vi "JSON DATA.vi"(0 "Temp Amb":refnum<class "JSON Object.lvclass">[](array[class]), 1 "Humedad R.":refnum<class "JSON Object.lvclass">[](array[class]), 2 "PAR":refnum<class "JSON Object.lvclass">[](array[class]), 3 "Numeric":i32, 5 "Temp Panel":refnum<class "JSON Object.lvclass">[](array[class]), 7 "Generador":refnum<class "JSON Object.lvclass">[](array[class]), 9 "JSON CARGA":refnum<class "JSON Array.lvclass">[](array[class]), 11 "error in":errorcluster, 12 "JSON FV":refnum<class "JSON Object.lvclass">[](array[class]), 13 "JSON BAT":refnum<class "JSON Object.lvclass">[](array[class]), 14 "alarmas":refnum<class "JSON Array.lvclass">[](array[class])) -> (4 "Array":refnum<class "JSON Object.lvclass">[](array[class]), 15 "error out":errorcluster)   [LabVIEW 2015]
uses:
  <vilib>/addons/JSON API/JSON Object/JSON Object.lvclass
  <vilib>/addons/JSON API/JSON Array/JSON Array.lvclass
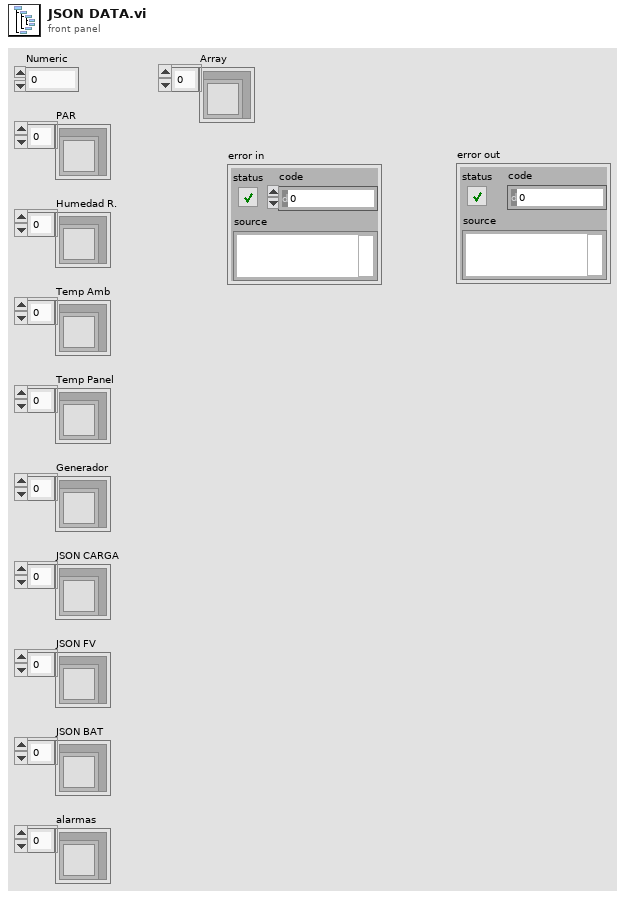
[diagram p1: front panel]
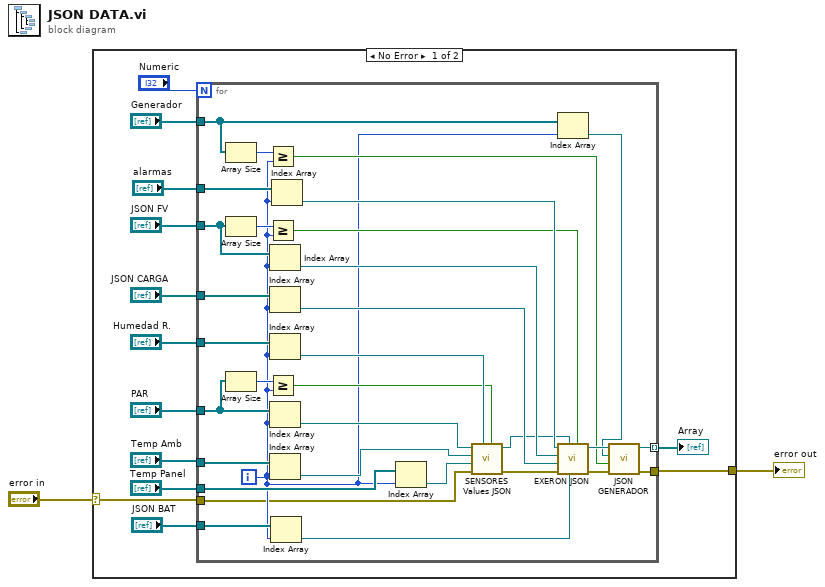
[diagram p0: block diagram]
diagram:
  n1 = case shown="No Error" "error in" {
    selector: "error in" -> [w5 w48]
    tunnel: [w4 w48] -> w1
    frame No Error {
      n2 = for {
        N: "Numeric" -> [_]
        tunnel: "PAR" -> [w38]
        tunnel: "Humedad R." -> [w39]
        tunnel: "Temp Amb" -> [w47]
        tunnel: "Temp Panel" -> [w46]
        tunnel: "JSON FV" -> [w28]
        tunnel: "JSON CARGA" -> [w37]
        tunnel: "JSON BAT" -> [w36]
        tunnel: "alarmas" -> [w35]
        tunnel: "Generador" -> [w21]
        tunnel: [w19] -> w15 mode=indexing
        tunnel: [w18] -> w4
        tunnel: w5 -> [w17]
        i -> [w20]
        n3 = Array Size(array=w21) -> (size(s)=w22:i32)
        n4 = Array Size(array=w28) -> (size(s)=w27:i32)
        n5 = Array Size(array=w38) -> (size(s)=w40:i32)
        n6 = Greater Or Equal?(x=w22, y=w20) -> (x >= y?=w23:bool)
        n7 = Greater Or Equal?(x=w27, y=w20) -> (x >= y?=w26:bool)
        n8 = Greater Or Equal?(x=w40, y=w20) -> (x >= y?=w41:bool)
        n9 = Index Array(array=w28, index=w20) -> (element=w34:refnum<class "JSON Object.lvclass">)
        n10 = Index Array(array=w37, index=w20) -> (element=w33:refnum<class "JSON Array.lvclass">)
        n11 = Index Array(array=w39, index=w20) -> (element=w44:refnum<class "JSON Object.lvclass">)
        n12 = Index Array(array=w38, index=w20) -> (element=w45:refnum<class "JSON Object.lvclass">)
        n13 = Index Array(array=w47, index=w20) -> (element=w43:refnum<class "JSON Object.lvclass">)
        n14 = Index Array(array=w36, index=w20) -> (element=w32:refnum<class "JSON Object.lvclass">)
        n15 = Index Array(array=w35, index=w20) -> (element=w31:refnum<class "JSON Array.lvclass">)
        n16 = Index Array(array=w46, index=w20) -> (element=w42:refnum<class "JSON Object.lvclass">)
        n17 = call "SENSORES Values JSON.vi"("Boolean"=w41, "JSON  HumeRel"=w44, "error in"=w17, "tempPanel"=w42, "tempAmb"=w43, "JSON PAR"=w45) -> ("error out"=w29:errorcluster, "JSON Object out"=w30:refnum<class "JSON Object.lvclass">)  [unwired: 4 in]
        n18 = Index Array(array=w21, index=w20) -> (element=w16:refnum<class "JSON Object.lvclass">)
        n19 = call "EXERON JSON.vi"("Boolean"=w26, "Baterias"=w32, "JSON Object in"=w30, "error in"=w29, "CARGA"=w33, "FV"=w34, "Alarmas"=w31) -> ("error out"=w24:errorcluster, "JSON Object out"=w25:refnum<class "JSON Object.lvclass">)  [unwired: 3 in]
        n20 = call "JSON GENERADOR.vi"("error in"=w24, "Boolean"=w23, "Value"=w16, "JSON Object in"=w25) -> ("error out"=w18:errorcluster, "JSON Object out"=w19:refnum<class "JSON Object.lvclass">)  [unwired: 6 in]
      }
      "Array" <- w15
    }
    frame Error {
    }
  }
  "error out" <- w1
